vi "SIRRectInCap.vi"(7 "outer a":dbl format="%.2f", 8 "P":cluster{"x":dbl, "y":dbl, "z":dbl}={"x"=1.0, "y"=-5.0, "z"=1.0} {"x" format="%.2f"; "z" format="%.2f"; "y" format="%.2f"}, 9 "Variables":T1={"sound spd (cm/s)"=150000, "time step (s)"=1e-09} {"time step (s)" format="%.2e"}, 11 "strip":cluster{"Radius":dbl, "h":dbl, "a":dbl}={"Radius"=10.0, "h"=3.0, "a"=5.0} {"Radius" format="%.2f"; "a" format="%.2f"; "h" format="%.2f"}) -> (1 "lower":dbl[](graph), 2 "upper":dbl[](graph), 3 "h rect":dbl[](graph), 4 "delay out":i32)   [LabVIEW 2022 SP3]
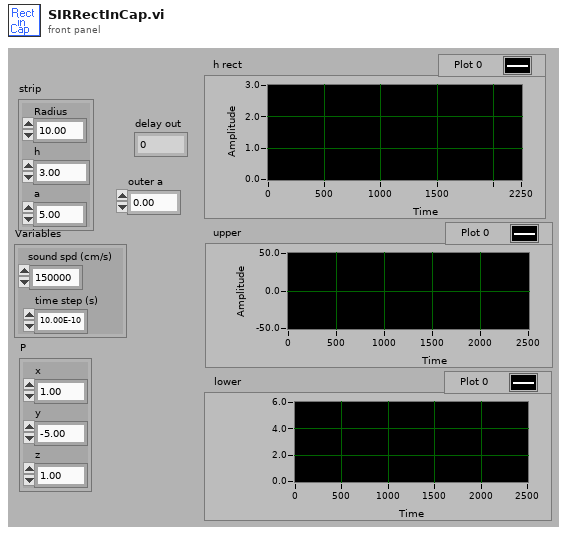
[diagram p1: front panel]
types:
  T1 = cluster{"sound spd (cm/s)":i32, "time step (s)":sgl}
  T2 = cluster{"Number of rings":i32, "sound spd (cm/s)":i32, "z span (cm)":dbl, "z steps":i32, "y span (cm)":dbl, "y steps":i32, "time step (s)":sgl, "z":dbl, "y":dbl, "ref delay":dbl, "freq (MHz)":dbl, "cycles":i32}
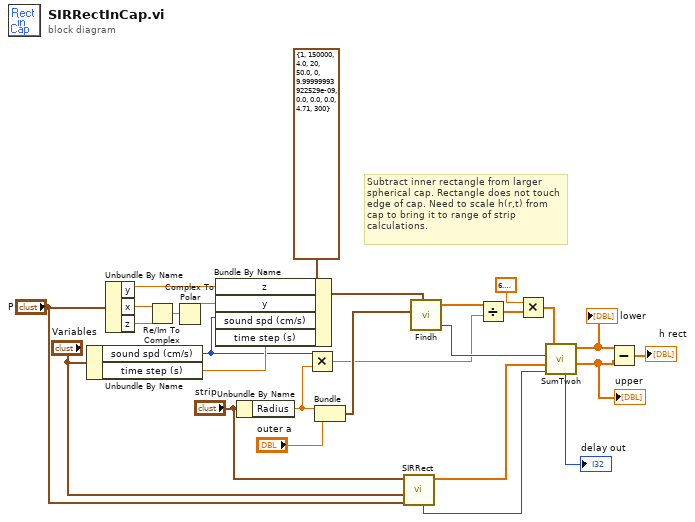
[diagram p0: block diagram]
diagram:
  # "Subtract inner rectangle from larger spherical cap. Rectangle does not touch edge of cap. Need to scale h(r,t) from cap to bring it to range of strip calculations."
  n1 = Unbundle By Name("Variables") -> ("sound spd (cm/s)"=w2:i32, "time step (s)"=w24:sgl)
  n2 = Unbundle By Name("P") -> ("y"=w22:dbl, "x"=w27:dbl, "z"=w26:dbl)
  n3 = Re/Im To Complex(1:w26, 2:w27) -> (0:w25:cdb)
  n4 = Complex To Polar(r * e^(i*theta)=w25) -> (r=w23:dbl)  [unwired: 1 out]
  n5 = Bundle By Name(cluster=T2 {"Number of rings"=1, "sound spd (cm/s)"=150000, "z span (cm)"=4.0, "z steps"=20, "y span (cm)"=50.0, "y steps"=0, "time step (s)"=1e-08, "z"=0.0, "y"=0.0, "ref delay"=0.0, "freq (MHz)"=4.71, "cycles"=300} ("Variables in"), "z"=w22, "y"=w23, "sound spd (cm/s)"=w2, "time step (s)"=w24) -> (w9:T2)
  n6 = Unbundle By Name("strip") -> ("Radius"=w1:dbl)
  n7 = Multiply(x=w2, y=w1) -> (x*y=w7:dbl)
  n8 = Bundle("Radius"=w1, "outer a"="outer a") -> (w19:cluster{"Radius":dbl, "outer a":dbl})  [unwired: 1 out]
  n9 = call "SIRRect.vi"("P"="P", "Variables"="Variables", "strip"="strip") -> ("h rect"=w14:dbl[], "delay out"=w13:i32)  [unwired: 7 out]
  n10 = call "Findh.vi"("Trans Geometry"=w19, "Variables in"=w9) -> ("h(r,t)"=w8:dbl[], "delay pts"=w15:i32)  [unwired: 1 in, 3 out]
  n11 = Divide(x=w8, y=w7) -> (x/y=w11:dbl[])
  n12 = Multiply(x=6.283185307179586, y=w11) -> (x*y=w6:dbl[])
  n13 = call "SumTwoh.vi"("h1"=w6, "delay1"=w15, "h2"=w14, "delay2"=w13) -> ("delay out"=→"delay out":i32, "upper"=w4:dbl[], "lower"=w3:dbl[])  [unwired: 2 out]
  "upper" <- w3
  "lower" <- w4
  n14 = Subtract(x=w4, y=w3) -> (x-y=→"h rect":dbl[])
